vi "ADC - Convert Integer to Floating Point Voltage.vi"(10 "Analog Integer Value In":i32) -> (2 "Analog Voltage (V)":dbl)   [LabVIEW 2021]
doc: "Converts an integer into a floating point value representing the voltage."
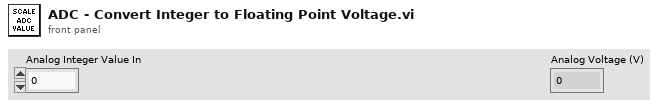
[diagram p1: front panel]
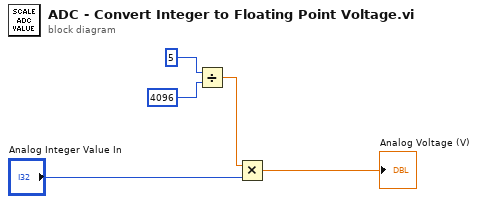
[diagram p0: block diagram]
diagram:
  n1 = Divide(x=5, y=4096) -> (x/y=w2:dbl)
  n2 = Multiply(x=w2, y="Analog Integer Value In") -> (x*y=→"Analog Voltage (V)":dbl)
